vi "Write.vi"(8 "error in (no error)":errorcluster, 9 "timeout_ms (-1)":i32=-1, 10 "Message":string, 11 "DETTWriter in":refnum<class "DETTWriter.lvclass">) -> (0 "error out":errorcluster, 3 "DETTWriter out":refnum<class "DETTWriter.lvclass">)   [LabVIEW 2024, in "DETTWriter.lvclass"]
uses:
  DETTWriter.lvclass
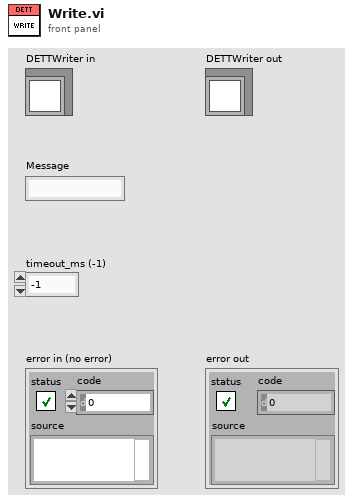
[diagram p1: front panel]
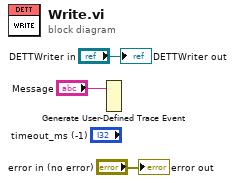
[diagram p0: block diagram]
diagram:
  n1 = Generate User-Defined Trace Event(2:"Message") -> ()  [unwired: 1 in]
  "error out" <- "error in (no error)"
  "DETTWriter out" <- "DETTWriter in"
